vi "getStatusBits.vi"(8 "error in (no error)":errorcluster, 10 "Axis Letter":string, 11 "Controller in":refnum<class "Controller.lvclass">) -> (0 "error out":errorcluster, 2 "StatusBits":T1, 3 "Controller out":refnum<class "Controller.lvclass">)   [LabVIEW 2019, in "Controller.lvclass"]
uses:
  Controller.lvclass
  Axis/Axis.lvclass
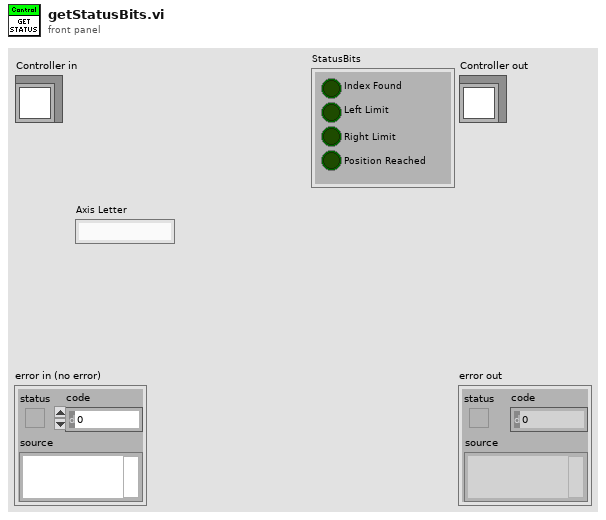
[diagram p1: front panel]
types:
  T1 = cluster{"Index Found":bool, "Left Limit":bool, "Right Limit":bool, "Position Reached":bool}
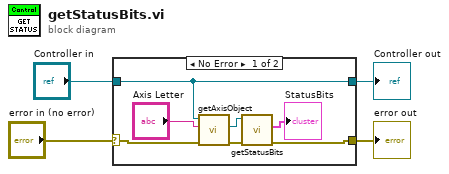
[diagram p0: block diagram]
diagram:
  n1 = case shown="No Error" "error in (no error)" {
    selector: "error in (no error)" -> [w9 w13]
    tunnel: [w6 w13] -> w3
    tunnel: [w11 w12] -> w1
    tunnel: "Controller in" -> [w11 w12]
    frame No Error {
      n2 = call-dynamic "getAxisObject.vi"("error in (no error)"=w9, "Axis Letter"="Axis Letter", "Controller in"=w11) -> ("error out"=w7:errorcluster, "Axis Object"=w8:refnum<class "Axis.lvclass">)  [unwired: 6 in, 1 out]
      n3 = call-dynamic "getStatusBits.vi"("error in (no error)"=w7, "Axis in"=w8) -> ("error out"=w6:errorcluster, "StatusBits"=→"StatusBits":T1)  [unwired: 7 in, 1 out]
    }
    frame Error {
    }
  }
  "error out" <- w3
  "Controller out" <- w1
